vi "Modify Existing Attribute Value.vi"(10 "Increment":T1, 11 "Value in":T1) -> (3 "Value out":T1)   [LabVIEW 2023]
doc: "This subVI modifies the existing attribute value."
uses:
  Lookup Table Data.ctl
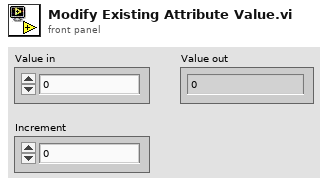
[diagram p1: front panel]
types:
  T1 = typedef "Lookup Table Data.ctl" = u32
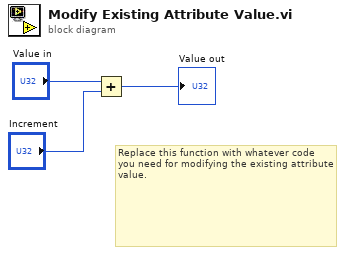
[diagram p0: block diagram]
diagram:
  # "Replace this function with whatever code you need for modifying the existing attribute value."
  n1 = Add(x="Value in", y="Increment") -> (x+y=→"Value out":T1)
